vi "MenuHandler.vi"(5 "tree control":refnum<vi>, 7 "main message queue":T1, 8 "error in":errorcluster, 9 "parameters":variant, 10 "menu string":string, 11 "RIO Target in":refnum<class "RIO Target.lvclass">) -> (0 "error out":errorcluster, 1 "refresh tree?":bool, 2 "Unhandled":bool, 3 "RIO Target out":refnum<class "RIO Target.lvclass">)   [LabVIEW 2014, in "RIO Target.lvclass"]
uses:
  RIO Target.lvclass
  <vilib>/NI/AMC/Message Queue.ctl
  <vilib>/NI/AMC/Message.ctl
  <vilib>/NI/Tools/Keyed Array/KeyedArray.ctl
  <vilib>/NI/AMC/Create Single Message.vi
  <vilib>/NI/AMC/Update Message Routing Info.vi
  <vilib>/NI/AMC/Send Message.vi
  <vilib>/NI/AMC/AMC.lvlib
  <vilib>/NI/Tools/Keyed Array/Tools_KeyedArray.lvlib
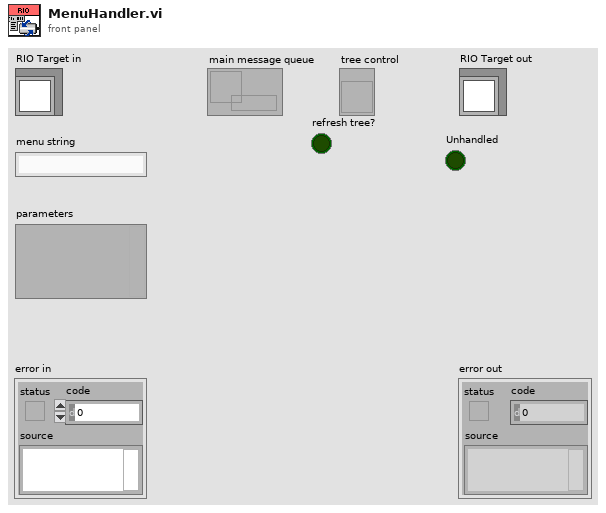
[diagram p1: front panel]
types:
  T1 = typedef "AMC.lvlib/Message Queue.ctl" = refnum<queue>
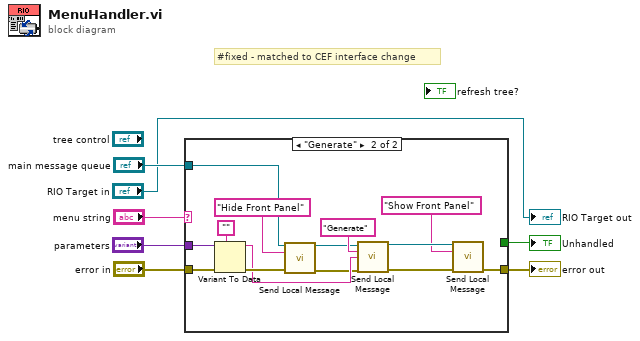
[diagram p0: block diagram]
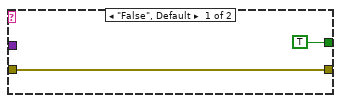
[diagram p2: hidden frame]
diagram:
  # "#fixed - matched to CEF interface change"
  n1 = case shown="\"Generate\"" "menu string" {
    tunnel: "parameters" -> [_ w13]
    tunnel: "error in" -> [w9 w12]
    tunnel: "main message queue" -> [_ w11]
    tunnel: [w9 w10] -> w2
    tunnel: [TRUE _] -> w1
    frame "False", Default {
    }
    frame "Generate" {
      n2 = Variant To Data(error in=w12, type="", Variant=w13) -> (data=w19:string, error out=w20:errorcluster)
      n3 = call <vilib>:"Send Local Message.vi"("message queue in"=w11, "message name"="Hide Front Panel", "error in"=w20) -> ("message queue out"=w15:T1, "error out"=w18:errorcluster)  [unwired: 10 in, 1 out]
      n4 = call <vilib>:"Send Local Message.vi"("message queue in"=w15, "message name"="Generate", "message value"=w19, "error in"=w18) -> ("message queue out"=w16:T1, "error out"=w17:errorcluster)  [unwired: 9 in, 1 out]
      n5 = call <vilib>:"Send Local Message.vi"("message queue in"=w16, "message name"="Show Front Panel", "error in"=w17) -> ("error out"=w10:errorcluster)  [unwired: 10 in, 2 out]
    }
  }
  "error out" <- w2
  "Unhandled" <- w1
  "RIO Target out" <- "RIO Target in"
